vi "set_config_cluster.vi"(8 "error in (no error)":errorcluster, 10 "config cluster variant":variant, 11 "AnalyserDL090623TwoD in":refnum<class "AnalyserDL090623TwoD.lvclass">) -> (0 "error out":errorcluster, 3 "AnalyserDL090623TwoD out":refnum<class "AnalyserDL090623TwoD.lvclass">)   [LabVIEW 2010, in "AnalyserDL090623TwoD.lvclass"]
uses:
  AnalyserDL090623TwoD.lvclass
  AnalyserDL090623TwoD.lvclass/AnalyserDL090623TwoD.ctl
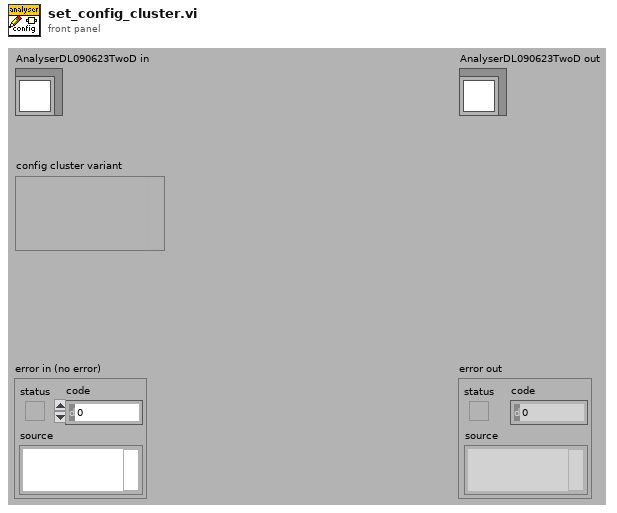
[diagram p1: front panel]
types:
  T1 = typedef "AnalyserDL090623TwoD.lvclass/config_data_cluster.ctl" = cluster{"segmenter":T2, "expression":string, "trace processor pipeline":T2[]}
  T2 = typedef "plugin_specification.ctl" = cluster{"class path":string, "configuration":string, "label":string, "settings name":string}
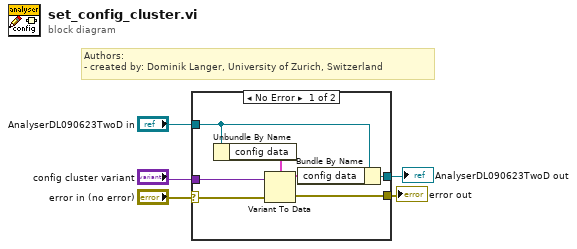
[diagram p0: block diagram]
diagram:
  # "Authors: \n- created by: Dominik Langer, University of Zurich, Switzerland"
  n1 = case shown="No Error" "error in (no error)" {
    selector: "error in (no error)" -> [w10 w13]
    tunnel: [w12 w13] -> w5
    tunnel: "config cluster variant" -> [w11 _]
    tunnel: "AnalyserDL090623TwoD in" -> [w8 w14]
    tunnel: [w6 w14] -> w1
    frame No Error {
      n2 = Unbundle By Name(w8) -> ("config data"=w9:T1)
      n3 = Variant To Data(error in=w10, Variant=w11, type=w9) -> (error out=w12:errorcluster, data=w7:T1)
      n4 = Bundle By Name(cluster=w8, "config data"=w7) -> (w6:refnum<class "AnalyserDL090623TwoD.lvclass">)
    }
    frame Error {
    }
  }
  "error out" <- w5
  "AnalyserDL090623TwoD out" <- w1
